vi "extract and prune to time range.vi"(8 "error in (no error)":errorcluster, 10 "time range":dbl, 11 "time and val queue":refnum<queue>) -> (0 "error out":errorcluster, 2 "graph":cluster{dbl[], dbl[]}, 3 "time and val queue out":refnum<queue>)   [LabVIEW 2017]
uses:
  typedefs/reading1.ctl
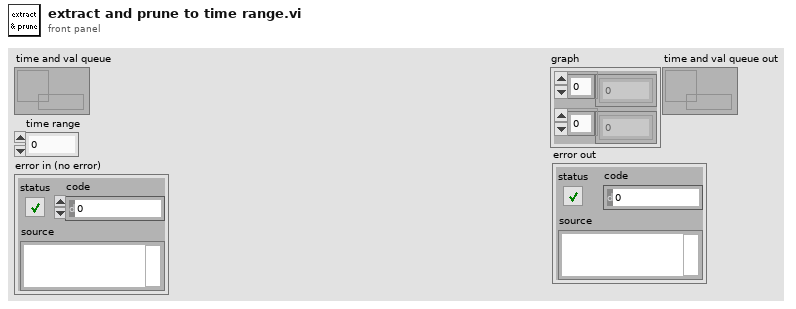
[diagram p1: front panel]
types:
  T1 = typedef "reading1.ctl" = cluster{"time":dbl, "x":dbl}
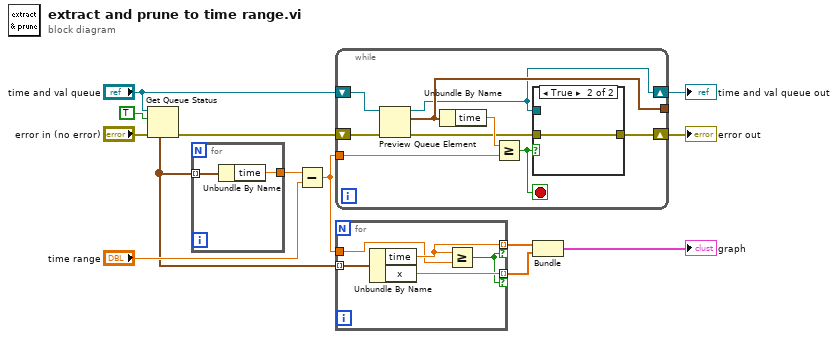
[diagram p0: block diagram]
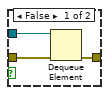
[diagram p2: hidden frame]
diagram:
  n1 = Get Queue Status(queue="time and val queue", return elements? (F)=TRUE, error in (no error)="error in (no error)") -> (error out=w10:errorcluster, elements=w8:T1[])  [unwired: 6 out]
  n2 = for {
    tunnel: w8 -> [w15] mode=indexing
    tunnel: [w14] -> w9
    n3 = Unbundle By Name(w15) -> ("time"=w14:dbl)
  }
  n4 = Subtract(x=w9, y="time range") -> (x-y=w7:dbl)
  n5 = while {
    tunnel: w7 -> [w21]
    shift-right: [w16] -> w2
    shift-left: w10 -> [w23]
    shift-right: [w18] -> w1
    shift-left: "time and val queue" -> [w24]
    tunnel: [w20] -> _
    stop <- w19 stop-if-true
    n6 = Preview Queue Element(queue=w24, error in (no error)=w23) -> (queue out=w18:refnum<queue>, element=w20:T1, error out=w17:errorcluster)  [unwired: 1 in, 1 out]
    n7 = Unbundle By Name(w20) -> ("time"=w22:dbl)
    n8 = Greater Or Equal?(x=w22, y=w21) -> (x >= y?=w19:bool)
    n9 = case shown="True" w19 {
      tunnel: w18 -> [w27 _]
      tunnel: w17 -> [w26 w28]
      tunnel: [w25 w28] -> w16
      frame False {
        n10 = Dequeue Element(queue=w27, error in (no error)=w26) -> (error out=w25:errorcluster)  [unwired: 1 in, 3 out]
      }
      frame True {
      }
    }
  }
  "error out" <- w2
  "time and val queue out" <- w1
  n11 = for {
    tunnel: w8 -> [w33] mode=indexing
    tunnel: [w31] -> w6 mode=indexing if=w29
    tunnel: [w32] -> w5 mode=indexing if=w29
    tunnel: w7 -> [w30]
    n12 = Unbundle By Name(w33) -> ("time"=w31:dbl, "x"=w32:dbl)
    n13 = Greater Or Equal?(x=w31, y=w30) -> (x >= y?=w29:bool)
  }
  n14 = Bundle(w6, w5) -> (→"graph":cluster{dbl[], dbl[]})  [unwired: 1 in]
